vi "运维调试_AADI5400.vi"() -> ()   [LabVIEW 2016, in "AADI5400.lvlib"]
uses:
  AADI5400.lvlib
  <vilib>/Instr/_visa.llb/VISA Configure Serial Port (Instr).vi
  <vilib>/Utility/config.llb/NI_LVConfig.lvlib
  <vilib>/ptbypt/NI_PtbyPt.lvlib
panel:
  out "通讯":bool
  in  "参数设置":bool
  out "显示":T1
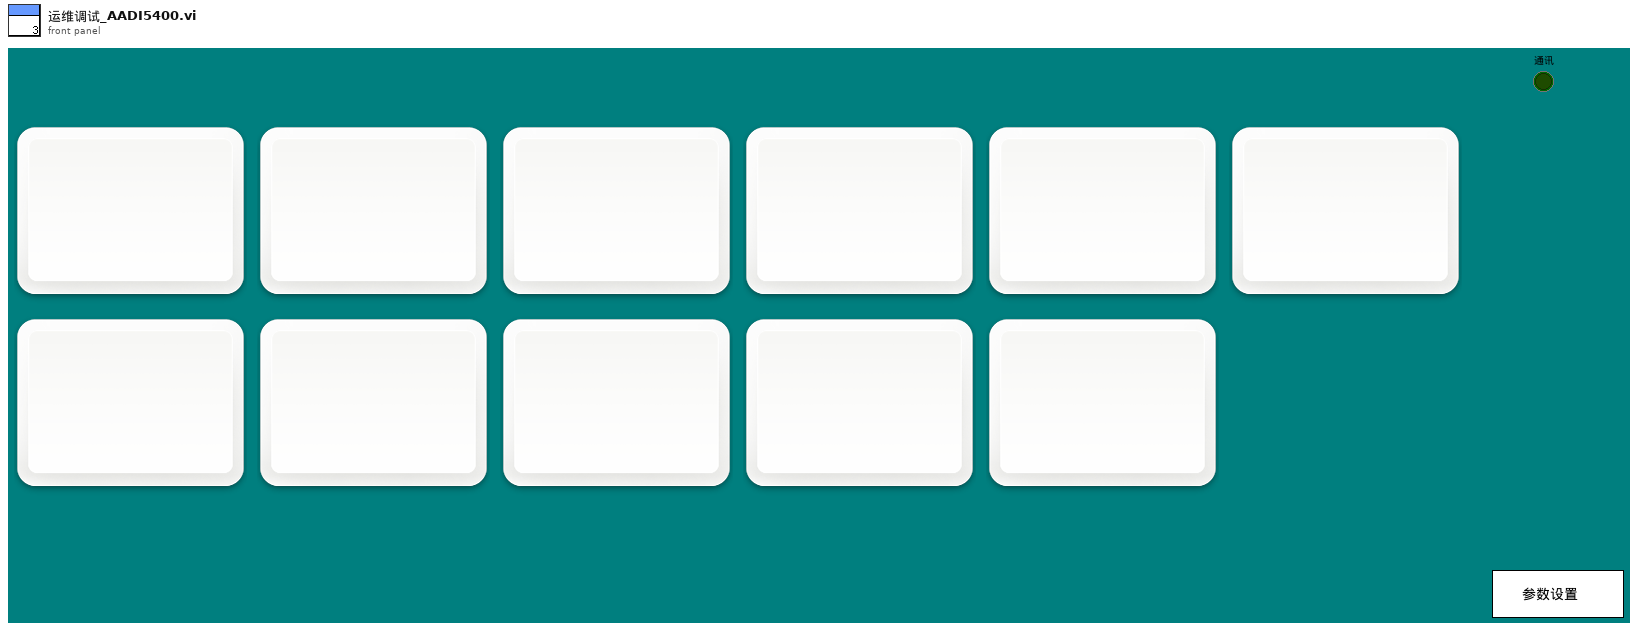
[diagram p1: front panel]
types:
  T1 = typedef "多数值显示.ctl" = cluster{"显示":T2, "显示 2":T2, "显示 3":T2, "显示 4":T2, "显示 5":T2, "显示 6":T2, "显示 12":T2, "显示 11":T2, "显示 10":T2, "显示 9":T2, "显示 8":T2, "显示 7":T2}
  T2 = typedef "数值显示.ctl" = cluster{"中文项目名称":string, "英文项目名称":string, "浓度":string, "单位":string}
  T3 = typedef "NI_LVConfig.lvlib/Config Data RefNum.ctl" = refnum<k1>
  T4 = typedef "LVDateTimeRec.ctl" = cluster{"秒数的小数部分":dbl, "秒":i32, "分":i32, "时":i32, "日":i32, "月":i32, "年":i32, "天数（周）":i32, "天数（年）":i32, "DST":i32}
  T5 = cluster{"seconds since 1Jan1904":timestamp, "浓度":string, "浓度":string, "浓度":string, "浓度":string, "浓度":string, "浓度":string, "浓度":string, "浓度":string, "浓度":string, "浓度":string, "浓度":string}
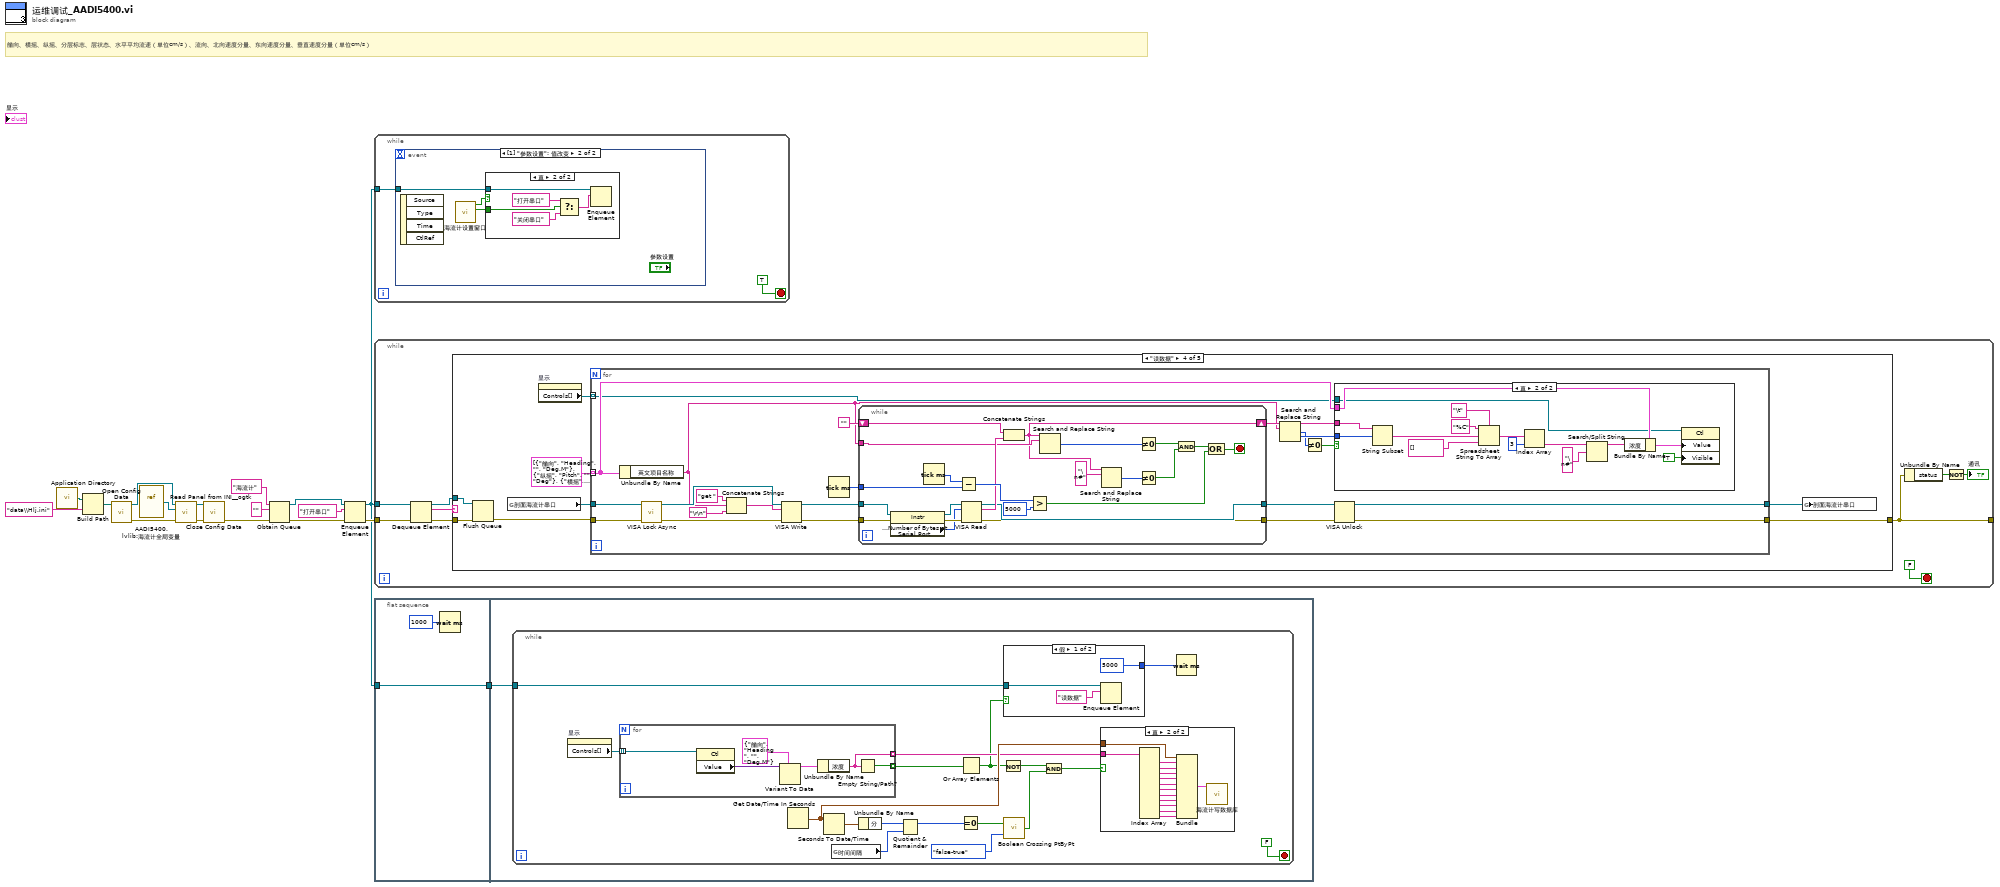
[diagram p0: block diagram]
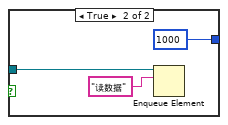
[diagram p3: hidden frame]
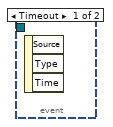
[diagram p4: hidden frame]
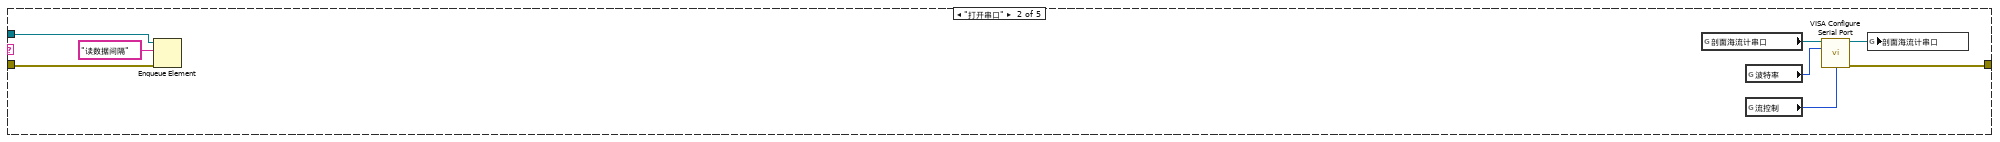
[diagram p7: hidden frame]
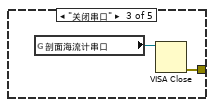
[diagram p8: hidden frame]
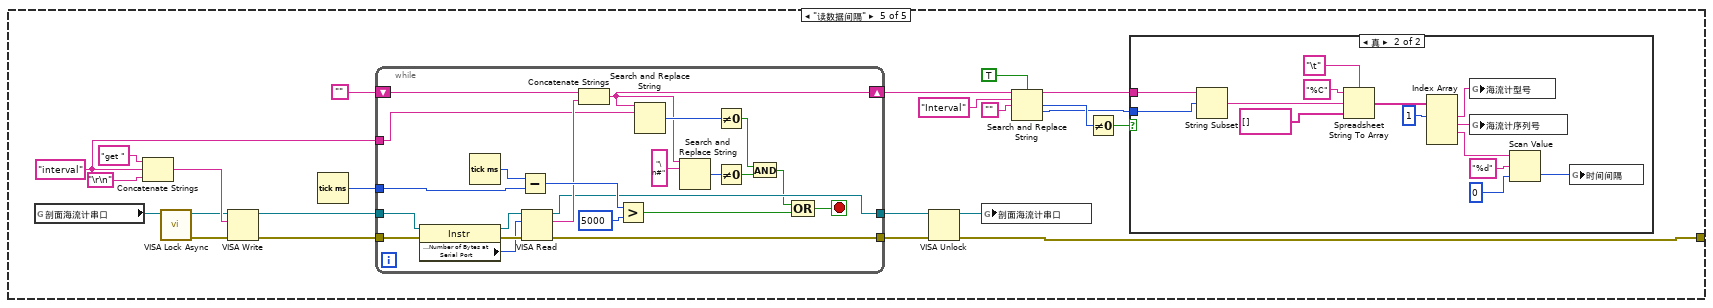
[diagram p10: hidden frame]
diagram:
  # "艏向、横摇、纵摇、分层标志、层状态、水平平均流速（单位cm/s）、流向、北向速度分量、东向速度分量、垂直速度分量（单位cm/s）"
  n1 = call <vilib>:"Application Directory.vi"() -> ("Application Directory"=w13:path)
  n2 = Build Path(base path=w13, name or relative path="data\\Hlj.ini" ("名称或相对路径")) -> (appended path=w15:path)
  n3 = call <vilib>:"Open Config Data.vi"("configuration file path"=w15) -> ("error out"=w11:errorcluster, "refnum"=w16:T3)  [unwired: 8 in, 1 out]
  n4 = vi-ref "AADI5400.lvlib:海流计全局变量.vi"() -> (w3:refnum<vi>)
  n5 = call <userlib>:"Read Panel from INI__ogtk.vi"("error in (no error)"=w11, "VI ref"=w3, "refnum"=w16) -> ("error out"=w12:errorcluster, "refnum out"=w17:T3)  [unwired: 7 in]
  n6 = call <vilib>:"Close Config Data.vi"("error in (no error)"=w12, "refnum"=w17) -> ("error out"=w8:errorcluster)  [unwired: 8 in, 1 out]
  n7 = Obtain Queue(name (unnamed)="海流计" ("名称（未命名）"), element data type="" ("状态"), error in (no error)=w8) -> (queue out=w5:refnum<queue>, error out=w6:errorcluster)  [unwired: 2 in, 1 out]
  n8 = Enqueue Element(queue=w5, element="打开串口" ("状态"), error in (no error)=w6) -> (queue out=w2:refnum<queue>, error out=w4:errorcluster)  [unwired: 1 in, 1 out]
  n9 = while {
    tunnel: w2 -> [w18]
    stop <- TRUE stop-if-true
    n10 = event shown="[1] \"参数设置\": 值改变" {
      selector: _ -> [_ _]
      dyn-events: _ -> [_ _]
      timeout: _ -> [_ _]
      tunnel: w18 -> [_ w20]
      event Timeout {
        n11 = event-data() -> ()  [unwired: 1 in, 3 out]
      }
      event "参数设置": Value Change {
        n12 = event-data() -> ()  [unwired: 1 in, 4 out]
        n13 = call "海流计设置窗口.vi"() -> ("开关"=w21:bool, "确定输出"=w22:bool)  [unwired: 10 in]
        n14 = case shown="真" w22 {
          tunnel: w21 -> [_ w27]
          tunnel: w20 -> [_ w23]
          frame False {
          }
          frame True {
            n15 = Select(t="打开串口" ("状态"), s=w27, f="关闭串口" ("状态")) -> (s? t:f=w24:string)
            n16 = Enqueue Element(queue=w23, element=w24) -> ()  [unwired: 2 in, 3 out]
          }
        }
      }
    }
  }
  n17 = while {
    tunnel: w2 -> [w36]
    tunnel: w4 -> [w35]
    tunnel: [w29] -> _
    stop <- FALSE stop-if-true
    n18 = Dequeue Element(queue=w36, error in (no error)=w35) -> (queue out=w32:refnum<queue>, element=w34:string, error out=w33:errorcluster)  [unwired: 1 in, 1 out]
    n19 = case shown="\"读数据\"" w34 {
      tunnel: w33 -> [w37 w40 _ w50 _]
      tunnel: [w37 w41 w46 w51 w125] -> w29
      tunnel: w32 -> [_ w39 _ w48 _]
      frame "假", Default {
      }
      frame "打开串口" {
        n20 = Enqueue Element(queue=w39, element="读数据间隔" ("元素"), error in (no error)=w40) -> ()  [unwired: 1 in, 3 out]
        n21 = global read "海流计全局变量.vi" "剖面海流计串口"() -> (w45:refnum<visa-resource-name>)
        n22 = global read "海流计全局变量.vi" "波特率"() -> (w44:u32)
        n23 = global read "海流计全局变量.vi" "流控制"() -> (w43:u16)
        n24 = call-poly "VISA Configure Serial Port"("VISA resource name"=w45, "baud rate (9600)"=w44, "flow control (0:none)"=w43) -> ("VISA resource name out"=w42:refnum<visa-resource-name>, "error out"=w41:errorcluster)  [unwired: 11 in]
        n25 = global write "海流计全局变量.vi" "剖面海流计串口"(w42) -> ()
      }
      frame "关闭串口" {
        n26 = global read "海流计全局变量.vi" "剖面海流计串口"() -> (w47:refnum<visa-resource-name>)
        n27 = VISA Close(VISA resource name=w47) -> (error out=w46:errorcluster)  [unwired: 1 in]
      }
      frame "读数据" {
        n28 = Flush Queue(queue=w48, error in (no error)=w50) -> (error out=w49:errorcluster)  [unwired: 2 out]
        n29 = global read "海流计全局变量.vi" "剖面海流计串口"() -> (w55:refnum<visa-resource-name>)
        n30 = property on="显示" class="Clust (严格)"() -> ("Controls[]"=w54:refnum<vi>[])  [unwired: 2 in, 2 out]
        n31 = for {
          tunnel: T2[] [{"中文项目名称"="艏向", "英文项目名称"="Heading", "浓度"="", "单位"="Deg.M"}, {"中文项目名称"="纵摇", "英文项目名称"="Pitch", "浓度"="", "单位"="Deg"}, {"中文项目名称"="横摇", "英文项目名称"="Roll", "浓度"="", "单位"="Deg"}, {"中文项目名称"="分层标志", "英文项目名称"="Cell Index", "浓度"="", "单位"=""}, {"中文项目名称"="层状态1", "英文项目名称"="Cell State1", "浓度"="", "单位"=""}, {"中文项目名称"="层状态2", "英文项目名称"="Cell State2", "浓度"="", "单位"=""}, {"中文项目名称"="水平平均流速", "英文项目名称"="Horizontal Speed", "浓度"="", "单位"="cm/s"}, {"中文项目名称"="流向", "英文项目名称"="Direction", "浓度"="", "单位"="Deg.M"}, {"中文项目名称"="北向流速分量", "英文项目名称"="North Speed", "浓度"="", "单位"="cm/s"}, {"中文项目名称"="东向流速分量", "英文项目名称"="East Speed", "浓度"="", "单位"="cm/s"}, {"中文项目名称"="垂直流速分量", "英文项目名称"="Vertical Speed", "浓度"="", "单位"="cm/s"}] -> [w63] mode=indexing
          tunnel: w55 -> [w72]
          tunnel: w49 -> [w71]
          tunnel: [w60] -> w52
          tunnel: [w59] -> w51
          tunnel: w54 -> [w56] mode=indexing
          n32 = Unbundle By Name(w63) -> ("英文项目名称"=w58:string)
          n33 = call <vilib>:"VISA Lock Async.vi"("error in (no error)"=w71, "VISA resource name"=w72) -> ("error out"=w69:errorcluster, "VISA resource name out"=w70:refnum<visa-resource-name>)  [unwired: 7 in, 1 out]
          n34 = Concatenate Strings("get ", w58, "\r\n") -> (w77:string)
          n35 = VISA Write(VISA resource name=w70, write buffer=w77, error in (no error)=w69) -> (VISA resource name out=w74:refnum<visa-resource-name>, error out=w73:errorcluster)  [unwired: 1 out]
          n36 = Tick Count (ms)() -> (millisecond timer value=w75:u32)
          n37 = while {
            tunnel: w74 -> [w116]
            tunnel: w73 -> [w115]
            tunnel: w75 -> [w109]
            shift-right: [w100] -> w68
            shift-left: "" -> [w107]
            tunnel: [w105] -> w62
            tunnel: [w104] -> w61
            tunnel: w58 -> [w101]
            stop <- w103 stop-if-true
            n38 = property class="Instr"(reference=w116, error in=w115) -> (reference out=w114:refnum<visa-resource-name>, error out=w113:errorcluster, "Serial Settings:Number of Bytes at Serial Port"=w112:u32)
            n39 = Tick Count (ms)() -> (millisecond timer value=w110:u32)
            n40 = Subtract(x=w110, y=w109) -> (x-y=w111:u32)
            n41 = VISA Read(VISA resource name=w114, byte count=w112, error in (no error)=w113) -> (VISA resource name out=w105:refnum<visa-resource-name>, read buffer=w106:string, error out=w104:errorcluster)  [unwired: 1 out]
            n42 = Concatenate Strings(w107, w106) -> (w100:string)
            n43 = Greater?(x=w111, y=u32 5000) -> (0:w97:bool)
            n44 = Search and Replace String(input string=w100, search string=w101) -> (number of replacements=w102:i32)  [unwired: 6 in, 3 out]
            n45 = Search and Replace String(input string=w100, search string="\n#") -> (number of replacements=w98:i32)  [unwired: 6 in, 3 out]
            n46 = Not Equal To 0?(x=w102) -> (x != 0?=w95:bool)
            n47 = Not Equal To 0?(x=w98) -> (x != 0?=w94:bool)
            n48 = And(x=w95, y=w94) -> (x .and. y?=w96:bool)
            n49 = Compound Arithmetic op=OR ("复合运算")(w96, w97) -> (w103:bool)
          }
          n50 = Search and Replace String(input string=w68, search string=w58) -> (result string=w67:string, number of replacements=w65:i32, offset past replacement=w66:i32)  [unwired: 6 in, 1 out]
          n51 = Not Equal To 0?(x=w65) -> (x != 0?=w64:bool)
          n52 = case shown="真" w64 {
            tunnel: w67 -> [_ w93]
            tunnel: w66 -> [_ w92]
            tunnel: w63 -> [_ w85]
            tunnel: w56 -> [_ w80]
            frame False {
            }
            frame True {
              n53 = String Subset(string=w93, offset (0)=w92) -> (substring=w91:string)  [unwired: 1 in]
              n54 = Spreadsheet String To Array(delimiter (Tab)="\t", format string="%C" ("格式字符串"), spreadsheet string=w91, array type (2D Dbl)=string[] []) -> (array=w87:string[])
              n55 = Index Array(array=w87, index=3 ("索引")) -> (element=w84:string)
              n56 = Search/Split String(string=w84, search string/char (-)="\n#") -> (substring before match=w82:string)  [unwired: 1 in, 2 out]
              n57 = Bundle By Name(cluster=w85, "浓度"=w82) -> (w79:T2)
              n58 = property class="Ctl"(reference=w80, "Value"=w79, "Visible"=TRUE ("可见")) -> ()  [unwired: 1 in, 2 out]
            }
          }
          n59 = VISA Unlock(8:w61, 11:w62) -> (0:w59:errorcluster, 3:w60:refnum<visa-resource-name>)
        }
        n60 = global write "海流计全局变量.vi" "剖面海流计串口"(w52) -> ()
      }
      frame "读数据间隔" {
        w129 = "interval" ("字符串")
        n61 = global read "海流计全局变量.vi" "剖面海流计串口"() -> (w134:refnum<visa-resource-name>)
        n62 = Concatenate Strings("get ", w129, "\r\n") -> (w138:string)
        n63 = call <vilib>:"VISA Lock Async.vi"("VISA resource name"=w134) -> ("error out"=w136:errorcluster, "VISA resource name out"=w137:refnum<visa-resource-name>)  [unwired: 8 in, 1 out]
        n64 = VISA Write(VISA resource name=w137, write buffer=w138, error in (no error)=w136) -> (VISA resource name out=w131:refnum<visa-resource-name>, error out=w130:errorcluster)  [unwired: 1 out]
        n65 = Tick Count (ms)() -> (millisecond timer value=w132:u32)
        n66 = while {
          tunnel: w131 -> [w176]
          tunnel: w130 -> [w175]
          tunnel: w132 -> [w169]
          shift-right: [w160] -> w117
          shift-left: "" -> [w167]
          tunnel: [w165] -> w128
          tunnel: [w164] -> w127
          tunnel: w129 -> [w161]
          stop <- w163 stop-if-true
          n67 = property class="Instr"(reference=w176, error in=w175) -> (reference out=w174:refnum<visa-resource-name>, error out=w173:errorcluster, "Serial Settings:Number of Bytes at Serial Port"=w172:u32)
          n68 = Tick Count (ms)() -> (millisecond timer value=w170:u32)
          n69 = Subtract(x=w170, y=w169) -> (x-y=w171:u32)
          n70 = VISA Read(VISA resource name=w174, byte count=w172, error in (no error)=w173) -> (VISA resource name out=w165:refnum<visa-resource-name>, read buffer=w166:string, error out=w164:errorcluster)  [unwired: 1 out]
          n71 = Concatenate Strings(w167, w166) -> (w160:string)
          n72 = Greater?(x=w171, y=u32 5000) -> (0:w157:bool)
          n73 = Search and Replace String(input string=w160, search string=w161) -> (number of replacements=w162:i32)  [unwired: 6 in, 3 out]
          n74 = Search and Replace String(input string=w160, search string="\n#") -> (number of replacements=w158:i32)  [unwired: 6 in, 3 out]
          n75 = Not Equal To 0?(x=w162) -> (x != 0?=w155:bool)
          n76 = Not Equal To 0?(x=w158) -> (x != 0?=w154:bool)
          n77 = And(x=w155, y=w154) -> (x .and. y?=w156:bool)
          n78 = Compound Arithmetic op=OR ("复合运算")(w156, w157) -> (w163:bool)
        }
        n79 = VISA Unlock(8:w127, 11:w128) -> (0:w125:errorcluster, 3:w126:refnum<visa-resource-name>)
        n80 = global write "海流计全局变量.vi" "剖面海流计串口"(w126) -> ()
        n81 = Search and Replace String(case sensitive?=TRUE ("忽略大小写？(F)"), input string=w117, search string="Interval" ("搜索字符串"), replace string="") -> (result string=w119:string, number of replacements=w122:i32, offset past replacement=w121:i32)  [unwired: 4 in, 1 out]
        n82 = Not Equal To 0?(x=w122) -> (x != 0?=w118:bool)
        n83 = case shown="真" w118 {
          tunnel: w121 -> [_ w153]
          tunnel: w119 -> [_ w152]
          frame False {
          }
          frame True {
            n84 = String Subset(string=w152, offset (0)=w153) -> (substring=w148:string)  [unwired: 1 in]
            n85 = Spreadsheet String To Array(delimiter (Tab)="\t", format string="%C" ("格式字符串"), spreadsheet string=w148, array type (2D Dbl)=string[] []) -> (array=w147:string[])
            n86 = Index Array(array=w147, index #1=1 ("索引")) -> (element #1=w145:string, element #2=w144:string, element #3=w143:string)  [unwired: 3 in, 1 out]
            n87 = global write "海流计全局变量.vi" "海流计型号"(w145) -> ()
            n88 = global write "海流计全局变量.vi" "海流计序列号"(w144) -> ()
            n89 = Scan Value(string=w143, format string="%d" ("格式字符串"), default (0 dbl)=u32 0) -> (value=w140:u32)  [unwired: 1 out]
            n90 = global write "海流计全局变量.vi" "时间间隔"(w140) -> ()
          }
        }
      }
    }
    n91 = Unbundle By Name(w29) -> ("status"=w30:bool)
    n92 = Not(x=w30) -> (.not. x?=→"通讯":bool)
  }
  n93 = flat-sequence {
    tunnel: w2 -> [w177]
    tunnel: [w177] -> w1
    tunnel: w1 -> [w179]
    frame #0 {
      n94 = Wait (ms)(milliseconds to wait=u32 1000 ("等待时间（毫秒）")) -> ()  [unwired: 1 out]
    }
    frame #1 {
      n95 = while {
        tunnel: w179 -> [w193]
        stop <- FALSE stop-if-true
        n96 = property on="显示" class="Clust (严格)"() -> ("Controls[]"=w196:refnum<vi>[])  [unwired: 2 in, 2 out]
        n97 = for {
          tunnel: w196 -> [w222] mode=indexing
          tunnel: [w218] -> w194 mode=indexing
          tunnel: [w217] -> w186 mode=indexing
          n98 = property class="Ctl"(reference=w222) -> ("Value"=w221:variant)  [unwired: 1 in, 2 out]
          n99 = Variant To Data(type=T2 {"中文项目名称"="艏向", "英文项目名称"="Heading", "浓度"="", "单位"="Deg.M"} ("显示 12"), Variant=w221) -> (data=w219:T2)  [unwired: 1 in, 1 out]
          n100 = Unbundle By Name(w219) -> ("浓度"=w217:string)
          n101 = Empty String/Path?(string/path=w217) -> (empty?=w218:bool)
        }
        n102 = Get Date/Time In Seconds() -> (seconds since 1Jan1904=w190:timestamp)
        n103 = Seconds To Date/Time(time stamp (now)=w190) -> (date time rec=w191:T4)  [unwired: 1 in]
        n104 = global read "海流计全局变量.vi" "时间间隔"() -> (w188:u32)
        n105 = Unbundle By Name(w191) -> ("分"=w189:i32)
        n106 = Quotient & Remainder(x=w189, y=w188) -> (x-y*floor(x/y)=w187:u32)  [unwired: 1 out]
        n107 = Or Array Elements(Boolean array=w194) -> (logical OR=w185:bool)
        n108 = Equal To 0?(x=w187) -> (x = 0?=w183:bool)
        n109 = Not(x=w185) -> (.not. x?=w184:bool)
        n110 = case shown="假" w185 {
          tunnel: w193 -> [w211 w216]
          tunnel: [u32 5000 ("等待时间（毫秒）") u32 1000 ("等待时间（毫秒）")] -> w192
          frame False {
            n111 = Enqueue Element(queue=w211, element="读数据" ("元素")) -> ()  [unwired: 2 in, 3 out]
          }
          frame True {
            n112 = Enqueue Element(queue=w216, element="读数据" ("元素")) -> ()  [unwired: 2 in, 3 out]
          }
        }
        n113 = call <vilib>:"Boolean Crossing PtByPt.vi"("direction"=enum16{"either", "false-true", "true-false"}."false-true", "input"=w183) -> ("crossing"=w181:bool)  [unwired: 1 in]
        n114 = And(x=w184, y=w181) -> (x .and. y?=w180:bool)
        n115 = case shown="真" w180 {
          tunnel: w190 -> [_ w198]
          tunnel: w186 -> [_ w197]
          frame False {
          }
          frame True {
            n116 = Index Array(array=w197) -> (element #1=w210:string, element #2=w209:string, element #3=w208:string, element #4=w207:string, element #5=w206:string, element #6=w205:string, element #7=w204:string, element #8=w203:string, element #9=w202:string, element #10=w201:string, element #11=w200:string)  [unwired: 11 in]
            n117 = Bundle("seconds since 1Jan1904"=w198, "浓度"=w210, "浓度"=w209, "浓度"=w208, "浓度"=w207, "浓度"=w206, "浓度"=w205, "浓度"=w204, "浓度"=w203, "浓度"=w202, "浓度"=w201, "浓度"=w200) -> (w199:T5)  [unwired: 1 in]
            n118 = call "海流计写数据库.vi"("data"=w199) -> ()  [unwired: 11 in]
          }
        }
        n119 = Wait (ms)(milliseconds to wait=w192) -> ()  [unwired: 1 out]
      }
    }
  }
